vi "ELVIS III v1.1 Open.vi"(8 "error in (no error)":errorcluster, 11 "Resource name":T2 caption="RIO Device") -> (0 "error out":errorcluster, 3 "myRIO FPGA Ref Out":T1)   [LabVIEW 2021]
uses:
  <vilib>/userDefined/High Color/nirio_resource_hc.ctl
  <vilib>/myRIO/Common/Instrument Driver Framework/Utilities/typedefs/Generic FPGA Reference.ctl
  <vilib>/myRIO/Common/Instrument Driver Framework/Utilities/typedefs/FPGA Ref Manager Action Enum.ctl
  <vilib>/myRIO/Common/Instrument Driver Framework/Utilities/typedefs/Ref Counter Action Enum.ctl
  <vilib>/FPGAPlugInAG/ELVIS III/niLvFpga_Open_ELVIS III.vi
  <vilib>/rvi/interface/common/dynamic/niFpgaDynamicAddResources.vi
  <vilib>/rvi/interface/nirviOpenFPGA/nirviOpenFPGA.xnode
  <vilib>/myRIO/FPGA/bitfiles/ELVIS III v1.1 FPGA.lvbitx
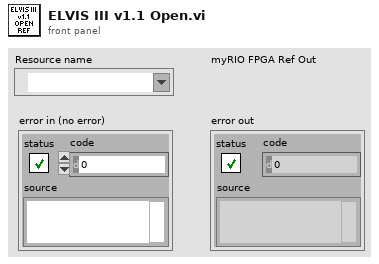
[diagram p1: front panel]
types:
  T1 = typedef "Generic FPGA Reference.ctl" = refnum<k20>
  T2 = typedef "nirio_resource_hc.ctl" = tag
  T3 = typedef "FPGA Ref Manager Action Enum.ctl" = enum16{"Get", "Set", "Reset"}
  T4 = typedef "Ref Counter Action Enum.ctl" = enum16{"Set", "Get", "Increment", "Decrement"}
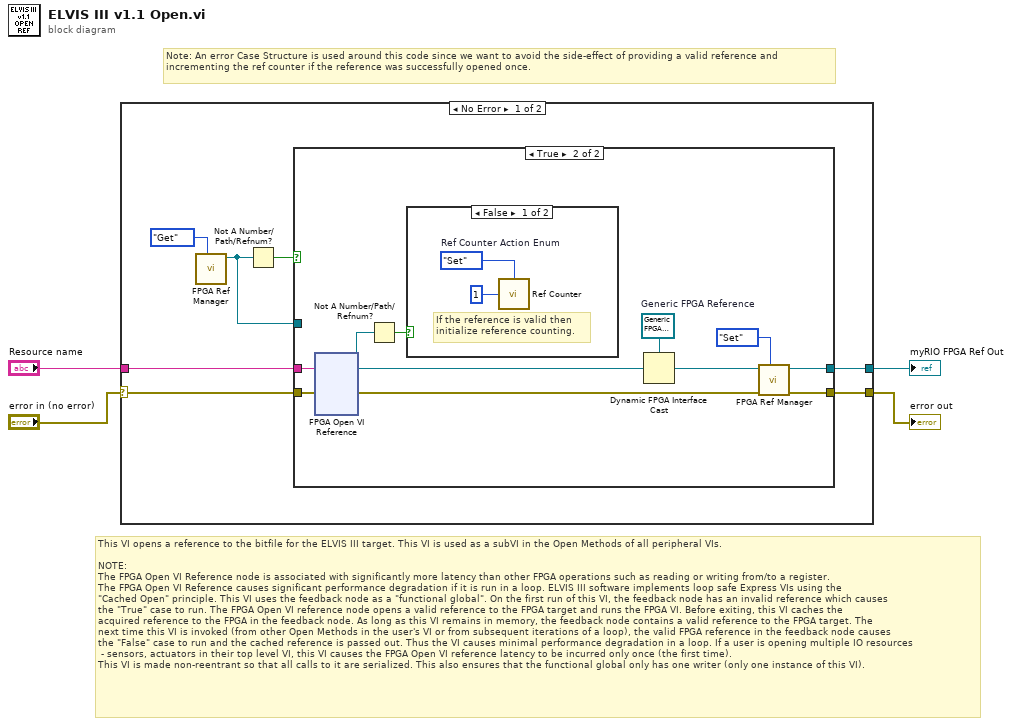
[diagram p0: block diagram]
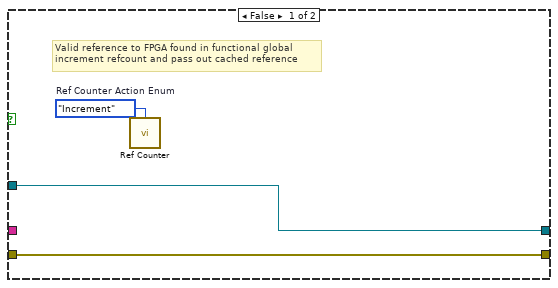
[diagram p2: hidden frame]
diagram:
  # "Note: An error Case Structure is used around this code since we want to avoid the side-effect of providing a valid reference and incrementing the ref counter if the reference was successfully opened once."
  # "This VI opens a reference to the bitfile for the ELVIS III target. This VI is used as a subVI in the Open Methods of all peripheral VIs.\n\nNOTE:\nThe FPGA Open VI Reference node is associated with significantly more latency than other FPGA operations such as reading or writing from/to a register. \nThe FPGA Open VI Reference causes significant performance degradation if it is run in a loop. ELVIS III software implements loop safe Express VIs using the \n\"Cached Open\" principle. This VI uses the feedback node as a \"functional global\". On the first run of this VI, the feedback node has an invalid reference which causes\nthe \"True\" case to run. The FPGA Open VI reference node opens a valid reference to the FPGA target and runs the FPGA VI. Before exiting, this VI caches the \nacquired reference to the FPGA in the feedback node. As long as this VI remains in memory, the feedback node contains a valid reference to the FPGA target. The \nnext time this VI is invoked (from other Open Methods in the user's VI or from subsequent iterations of a loop), the valid FPGA reference in the feedback node causes \nthe \"False\" case to run and the cached reference is passed out. Thus the VI causes minimal performance degradation in a loop. If a user is opening multiple IO resources\n - sensors, actuators in their top level VI, this VI causes the FPGA Open VI reference latency to be incurred only once (the first time).\nThis VI is made non-reentrant so that all calls to it are serialized. This also ensures that the functional global only has one writer (only one instance of this VI)."
  n1 = case shown="No Error" "error in (no error)" {
    selector: "error in (no error)" -> [w8 w27]
    tunnel: "Resource name" -> [w11 _]
    tunnel: [w10 _] -> w1
    tunnel: [w9 w27] -> w2
    frame No Error {
      n2 = call <vilib>:"FPGA Ref Manager.vi"("Action"=FPGA_Ref_Manager_Action_Enum."Get") -> ("Generic FPGA Reference out"=w6:T1)  [unwired: 8 in, 1 out]
      n3 = Not A Number/Path/Refnum?(number/path/refnum=w6) -> (NaN/Path/Refnum?=w7:bool)
      n4 = case shown="True" w7 {
        tunnel: w11 -> [_ w20]
        tunnel: w8 -> [w13 w19]
        tunnel: [w13 w22] -> w9
        tunnel: [w14 w23] -> w10
        tunnel: w6 -> [w14 _]
        frame False {
          w12 = Ref_Counter_Action_Enum."Increment"  # Ref Counter Action Enum
          # "Valid reference to FPGA found in functional global\nincrement refcount and pass out cached reference"
          n5 = call <vilib>:"Ref Counter.vi"("Ref Counter Action Enum"=w12) -> ()  [unwired: 1 in, 1 out]
        }
        frame True {
          w17 = T1 refnum  # Generic FPGA Reference
          n6 = xnode ("FPGA Open VI Reference")("error in"=w19, "resource name"=w20) -> ("FPGA VI Reference Out"=w16:refnum<k20>, "error out"=w15:errorcluster)
          n7 = Not A Number/Path/Refnum?(number/path/refnum=w16) -> (NaN/Path/Refnum?=w24:bool)
          n8 = case shown="False" w24 {
            frame False {
              w25 = Ref_Counter_Action_Enum."Set"  # Ref Counter Action Enum
              # "If the reference is valid then initialize reference counting."
              n9 = call <vilib>:"Ref Counter.vi"("Ref Count in"=u32 1 ("RefCount in"), "Ref Counter Action Enum"=w25) -> ()  [unwired: 1 out]
            }
            frame True {
              # "No error is thrown since the error will be generated by the Open node."
            }
          }
          n10 = Dynamic FPGA Interface Cast(Session In=w17, Type=w16) -> (Session Out=w18:T1)
          n11 = call <vilib>:"FPGA Ref Manager.vi"("Action"=FPGA_Ref_Manager_Action_Enum."Set", "error in (no error)"=w15, "Generic FPGA Reference in"=w18) -> ("error out"=w22:errorcluster, "Generic FPGA Reference out"=w23:T1)  [unwired: 6 in]
        }
      }
    }
    frame Error {
    }
  }
  "error out" <- w2
  "myRIO FPGA Ref Out" <- w1
